vi "Set - Matrix - Complex.vi"(8 "error in":errorcluster, 9 "value":cdb[][](array[numeric]), 10 "variable name":string, 11 "pipe in":T1) -> (0 "error out":errorcluster, 3 "pipe out":T1)   [LabVIEW 2013, in "GOLPI library.lvlib"]
uses:
  GOLPI library.lvlib
  LV Process.lvlibp/Pipe Handle.ctl
  Globals.vi
  LV Process.lvlibp
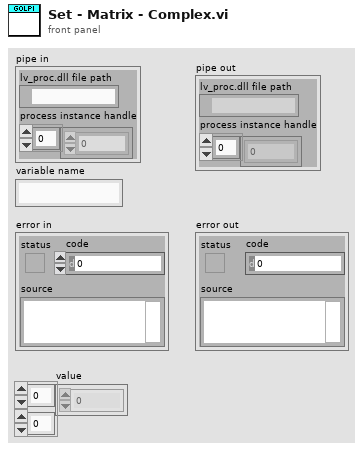
[diagram p1: front panel]
types:
  T1 = typedef "LV Process.lvlibp/Pipe Handle.ctl" = cluster{"lv_proc.dll file path":path, "process instance handle":u32[]}
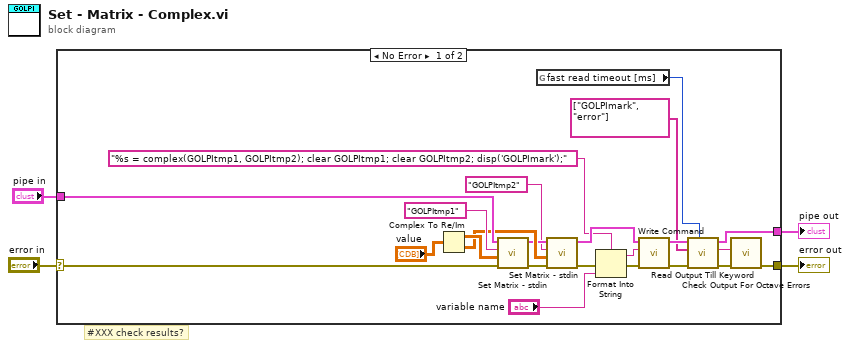
[diagram p0: block diagram]
diagram:
  # "#XXX check results?"
  n1 = case shown="No Error" "error in" {
    selector: "error in" -> [w27 w29]
    tunnel: [w12 w29] -> w4
    tunnel: "pipe in" -> [w26 w28]
    tunnel: [w15 w28] -> w1
    frame No Error {
      n2 = Complex To Re/Im(x + iy="value") -> (x=w24:dbl[][], y=w22:dbl[][])
      n3 = call "Set Matrix - stdin.vi"("error in"=w27, "value"=w24, "variable name"="GOLPItmp1", "pipe in"=w26) -> ("error out"=w20:errorcluster, "pipe out"=w21:T1)  [unwired: 6 in]
      n4 = global read "Globals.vi" "fast read timeout [ms]"() -> (w11:u32)
      n5 = call "Set Matrix - stdin.vi"("error in"=w20, "value"=w22, "variable name"="GOLPItmp2", "pipe in"=w21) -> ("error out"=w8:errorcluster, "pipe out"=w18:T1)  [unwired: 6 in]
      n6 = Format Into String(format string="%s = complex(GOLPItmp1, GOLPItmp2); clear GOLPItmp1; clear GOLPItmp2; disp('GOLPImark');" ("command"), error in=w8, "variable name") -> (resulting string=w5:string, error out=w7:errorcluster)  [unwired: 1 in]
      n7 = call "Write Command.vi"("error in"=w7, "command"=w5, "pipe in"=w18) -> ("error out"=w6:errorcluster, "pipe out"=w17:T1)  [unwired: 7 in]
      n8 = call "Read Output Till Keyword.vi"("timeout [ms]"=w11, "error in"=w6, "keywords"=string[] ["GOLPImark", "error"], "pipe in"=w17) -> ("error out"=w13:errorcluster, "read buffer"=w14:string, "pipe out"=w15:T1)  [unwired: 4 in, 1 out]
      n9 = call "Check Output For Octave Errors.vi"("error in"=w13, "read buffer"=w14) -> ("error out"=w12:errorcluster)  [unwired: 9 in]
    }
    frame Error {
    }
  }
  "error out" <- w4
  "pipe out" <- w1
